vi "Acc_reat from past data.vi"() -> ()   [LabVIEW 2020]
uses:
  <vilib>/ptbypt/NI_PtbyPt.lvlib
panel:
  out "Xaxis Signals":dynamicdata(graph)
  out "Motor":bool
  in  "Motor Enable":bool
  out "First Peak":bool
  out "peak 2":bool
  out "peak 1":bool
  in  "threshold":dbl(slide) scale=-15.0..15.0
  in  "Width":i32(slide)=10 min=3 scale=3.0..20.0
  out "Filtered \nSignal 2":dynamicdata(graph) caption="Filtered Signal"
  in  "Record Signal":bool
  out "Raw Voltage Output":dynamicdata(graph) caption="Raw Voltage Output Dx"
  in  "STOP":bool
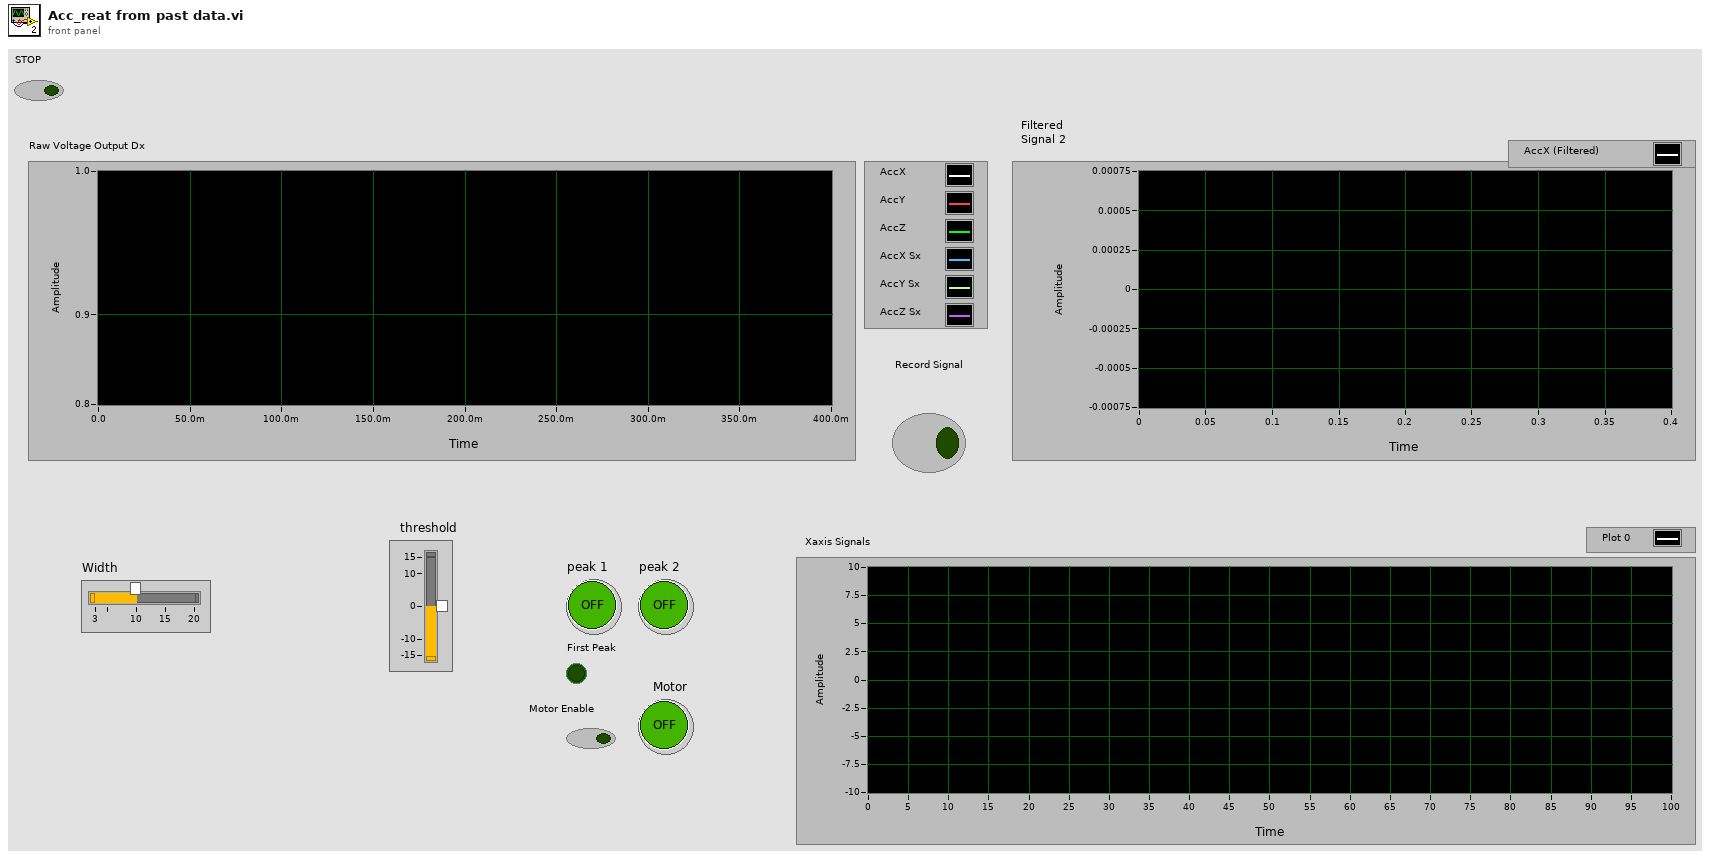
[diagram p1: front panel]
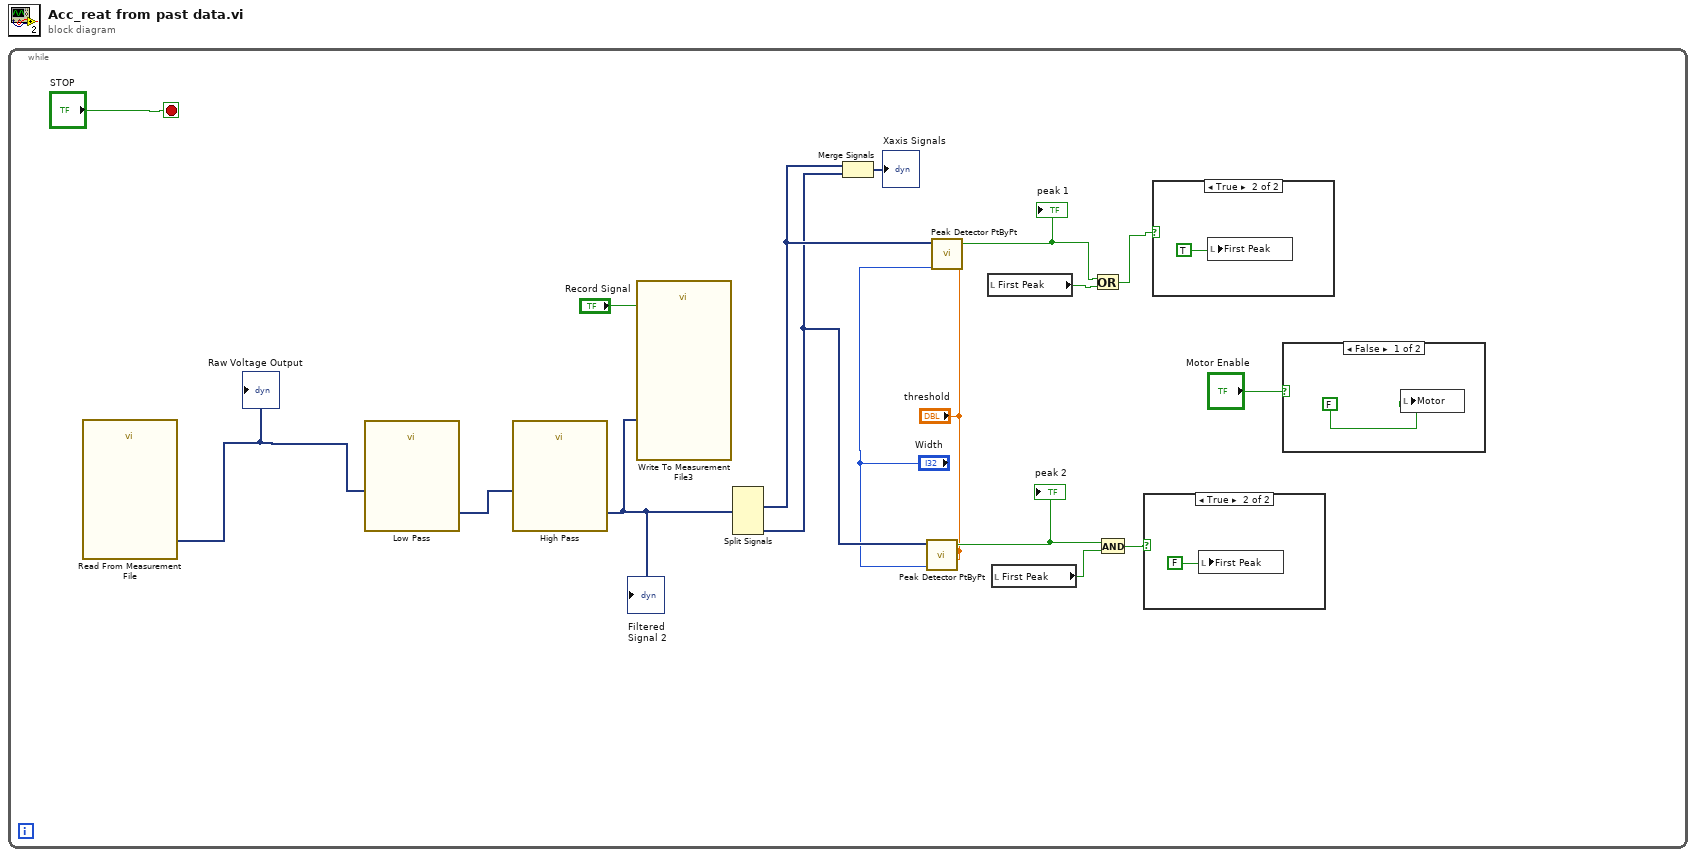
[diagram p0: block diagram]
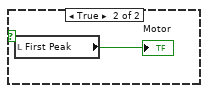
[diagram p2: hidden frame]
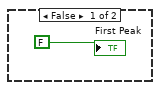
[diagram p4: hidden frame]
diagram:
  n1 = while {
    stop <- "STOP" stop-if-true
    n2 = call "Read From Measurement File"() -> ("Signals"=w2:dynamicdata)  [unwired: 6 in, 5 out]
    "Raw Voltage Output" <- w2
    n3 = call "Low Pass"("Signal"=w2) -> ("Filtered Signal"=w16:dynamicdata)  [unwired: 9 in, 1 out]
    n4 = call "High Pass"("Signal"=w16) -> ("Filtered Signal"=w14:dynamicdata)  [unwired: 9 in, 1 out]
    "Filtered \nSignal 2" <- w14
    n5 = call "Write To Measurement File3"("Signals"=w14, "Enable"="Record Signal") -> ()  [unwired: 15 in, 3 out]
    n6 = Split Signals(w14) -> (w6:dynamicdata, w5:dynamicdata)  [unwired: 6 in, 4 out]
    n7 = Merge Signals(w6, w5) -> (→"Xaxis Signals":dynamicdata)
    n8 = call <vilib>:"Peak Detector PtByPt.vi"("x"=w5, "threshold peak"="threshold", "threshold valley"="threshold", "width"="Width") -> ("peak"=w11:bool)  [unwired: 1 in, 2 out]
    "peak 2" <- w11
    n9 = call <vilib>:"Peak Detector PtByPt.vi"("x"=w6, "threshold peak"="threshold", "threshold valley"="threshold", "width"="Width") -> ("peak"=w8:bool)  [unwired: 1 in, 2 out]
    "peak 1" <- w8
    n10 = local read "First Peak"() -> (w7:bool)
    n11 = local read "First Peak"() -> (w10:bool)
    n12 = Or(x=w8, y=w7) -> (x .or. y?=w9:bool)
    n13 = And(x=w11, y=w10) -> (x .and. y?=w12:bool)
    n14 = case shown="True" w12 {
      frame False {
      }
      frame True {
        n15 = local write "First Peak"(FALSE) -> ()
      }
    }
    n16 = case shown="True" w9 {
      frame False {
        "First Peak" <- FALSE
      }
      frame True {
        n17 = local write "First Peak"(TRUE) -> ()
      }
    }
    n18 = case shown="False" "Motor Enable" {
      frame False {
        n19 = local write "Motor"(FALSE) -> ()
      }
      frame True {
        n20 = local read "First Peak"() -> (→"Motor":bool)
      }
    }
  }
